vi "OAT Order Cross Spectrum (1x1).vi"(0 "even-angle signal X":cluster{"r0":dbl, "dr":dbl, "Y":dbl[]}={"r0"=0.0, "dr"=1.0, "Y"=[]} {"r0" format="%.2p"; "dr" format="%.2p"; "Y" format="%.2f"}, 1 "even-angle signal Y":cluster{"r0":dbl, "dr":dbl, "Y":dbl[]}={"r0"=0.0, "dr"=1.0, "Y"=[]} {"r0" format="%.2p"; "dr" format="%.2p"; "Y" format="%.2f"}, 2 "window":u32(ring)=1 items=["None"=0, "Hanning"=1, "Hamming"=2, "Blackman-Harris"=3, "Exact Blackman"=4, "Blackman"=5, "Flat Top"=6, "4 Term B-Harris"=7, "7 Term B-Harris"=8, "Low Sidelobe"=9, "Gaussian"=62], 3 "block size":i32=1024 min=2, 4 "view":T6={"dB On (T)"=TRUE, "unwrap phase (F)"=FALSE, "convert to degree (T)"=TRUE}, 5 "error in (no error)":errorcluster, 6 "even-angle channel info X":T1={"channel name"="", "description"="", " channel info"={"sensor sensitivity"=1000.0, "engineering units"=1, "dB reference"=1.0, "custom label"="EU", "weighting filter"=0, "pregain"=0.0}} {"channel info"."pregain" format="%.2f"; "channel info"."weighting filter" items=["Linear", "A-weighting", "B-weighting", "C-weighting", "ITU-R 468-4", "Dolby", "CCITT", "C-message", "Wb", "Wc", "Wd", "We", "Wf", "Wh", "Wj", "Wk", "Wm", "AES17 20 kHz lowpass", "AES17 40 kHz lowpass", "AES17 20 kHz highpass", "AES17 40 kHz highpass"]; "channel info"."dB reference" format="%^.1e"; "channel info"."engineering units" items=["custom..."=0, "V"=1, "A"=21, "C"=30, "pC"=31, "s"=32, "-"=29, "Pa"=2, "N"=20, "g"=3, "m/s^2"=4, "m/s"=5, "m"=6, "mm/s"=12, "mm"=13, "micron/s"=14, "micron"=15, "in/s^2"=7, "in/s"=8, "in"=9, "mil/s"=10, "mil"=11, "rad/s^2"=16, "rad/s"=17, "rad"=18, "deg/s^2"=26, "deg/s"=27, "deg"=28, "RPM"=22, "cycle/s^2"=23, "Hz"=24, "cycle"=25, "strain"=19]; "channel info"."sensor sensitivity" format="%#_5f"}, 7 "averaging parameters":T11={"averaging mode"=enum."No averaging", "weighting mode"=enum."Exponential", "number of averages"=10, "linear mode"=enum."One shot"} {"number of averages" min=1 step=1}, 8 "even-angle channel info Y":T1={"channel name"="", "description"="", " channel info"={"sensor sensitivity"=1000.0, "engineering units"=1, "dB reference"=1.0, "custom label"="EU", "weighting filter"=0, "pregain"=0.0}} {"channel info"."pregain" format="%.2f"; "channel info"."weighting filter" items=["Linear", "A-weighting", "B-weighting", "C-weighting", "ITU-R 468-4", "Dolby", "CCITT", "C-message", "Wb", "Wc", "Wd", "We", "Wf", "Wh", "Wj", "Wk", "Wm", "AES17 20 kHz lowpass", "AES17 40 kHz lowpass", "AES17 20 kHz highpass", "AES17 40 kHz highpass"]; "channel info"."dB reference" format="%^.1e"; "channel info"."engineering units" items=["custom..."=0, "V"=1, "A"=21, "C"=30, "pC"=31, "s"=32, "-"=29, "Pa"=2, "N"=20, "g"=3, "m/s^2"=4, "m/s"=5, "m"=6, "mm/s"=12, "mm"=13, "micron/s"=14, "micron"=15, "in/s^2"=7, "in/s"=8, "in"=9, "mil/s"=10, "mil"=11, "rad/s^2"=16, "rad/s"=17, "rad"=18, "deg/s^2"=26, "deg/s"=27, "deg"=28, "RPM"=22, "cycle/s^2"=23, "Hz"=24, "cycle"=25, "strain"=19]; "channel info"."sensor sensitivity" format="%#_5f"}, 9 "restart averaging? (F)":bool) -> (11 "averaging done?":bool, 12 "new spectrum available?":bool, 13 "averages completed":dbl, 14 "cross spectrum magnitude":T5={"order 0"=0.0, "delta order"=1.0, "magnitude"=[]} {"order 0" format="%.2p"; "delta order" format="%.2p"; "magnitude" format="%.2f"}, 15 "magnitude unit label":string, 16 "cross spectrum phase":T5={"order 0"=0.0, "delta order"=1.0, "magnitude"=[]} {"order 0" format="%.2p"; "delta order" format="%.2p"; "magnitude" format="%.2f"}, 17 "phase unit label":string, 18 "spectrum info":T7={"channel name"="", "description"="", "x-axis units"=0, "spectral info"={"spectrum type"=enum."Power [Magnitude^2]", "linear/dB"=enum."linear", "window"=0, "window size"=0, "FFT size"=0}, "engineering units"=1, "custom label"="", "dB reference [EU]"=0.0, "peak units"=enum."rms", "weighting filter"=0, "spectral density?"=FALSE, "unit label"="", "spectrum skewed?"=FALSE, "complimentary spectrum units"=enum."none"} {"x-axis units" items=["Time (s)"=0, "Frequency-CB (Hz)"=1, "Frequency-CPB (Hz)"=1248, "Frequency-Arbitrary (Hz)"=2357, "Quefrency (s)"=2, "Revolutions (rev)"=3, "Order"=4, "Speed (RPM)"=11, "Speed (rad/s)"=21, "Index"=65535]; "weighting filter" items=["Linear", "A-weighting", "B-weighting", "C-weighting", "ITU-R 468-4", "Dolby", "CCITT", "C-message", "Wb", "Wc", "Wd", "We", "Wf", "Wh", "Wj", "Wk", "Wm", "AES17 20 kHz lowpass", "AES17 40 kHz lowpass", "AES17 20 kHz highpass", "AES17 40 kHz highpass"]; "dB reference [EU]" format="%.2f"; "engineering units" items=["custom..."=0, "V"=1, "A"=21, "C"=30, "pC"=31, "s"=32, "-"=29, "Pa"=2, "N"=20, "g"=3, "m/s^2"=4, "m/s"=5, "m"=6, "mm/s"=12, "mm"=13, "micron/s"=14, "micron"=15, "in/s^2"=7, "in/s"=8, "in"=9, "mil/s"=10, "mil"=11, "rad/s^2"=16, "rad/s"=17, "rad"=18, "deg/s^2"=26, "deg/s"=27, "deg"=28, "RPM"=22, "cycle/s^2"=23, "Hz"=24, "cycle"=25, "strain"=19]; "spectral info"."window" items=["None "=0, "Hanning"=1, "Hamming"=2, "Blackman-Harris"=3, "Exact Blackman"=4, "Blackman"=5, "Flat Top"=6, "4 Term B-Harris "=7, "7 Term B-Harris"=8, "Low Sidelobe"=9, "Force - Exponential"=10, "Gaussian"=62]}, 19 "error out":errorcluster)   [LabVIEW 2017, in "SoundVib_OrderTracking.lvlib"]
doc: "Computes the order power spectrum of an even-angle signal. Wire data to the <B>even-angle signal</B> input to determine the polymorphic instance to use or manually select the instance."
uses:
  <vilib>/addons/Sound and Vibration/Order Analysis/Resample Order Tracking/SoundVib_OrderTracking.lvlib
  <vilib>/addons/_NISVFA/_Shared subVIs/Controls/svc_Spectrum Info.ctl
  <vilib>/addons/_NISVFA/_Shared subVIs/Controls/svc_X-Axis Units.ctl
  <vilib>/addons/_NISVFA/_Shared subVIs/Controls/svc_Spectrum Type.ctl
  <vilib>/addons/_NISVFA/_Shared subVIs/Controls/svc_Engineering Units Text Ring.ctl
  <vilib>/addons/_NISVFA/_Shared subVIs/Controls/svc_Weighting Filter Text Ring.ctl
  <vilib>/addons/_NISVFA/_Shared subVIs/Controls/svc_Complimentary Spectrum Units.ctl
  <vilib>/addons/_NISVFA/_Shared subVIs/Controls/svc_Resampled Channel Info.ctl
  <vilib>/addons/_NISVFA/_Shared subVIs/Controls/svc_Channel Info.ctl
  <vilib>/addons/Sound and Vibration/Order Analysis/Resample Order Tracking/SoundVib_Resampling.lvlib
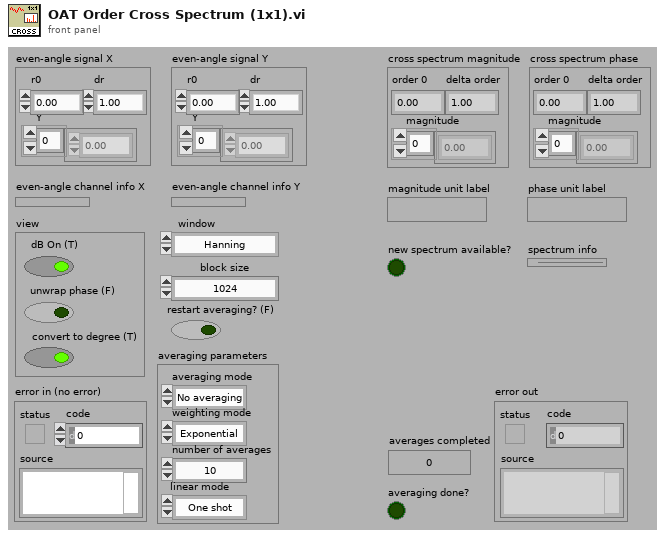
[diagram p1: front panel]
types:
  T1 = typedef "svc_Resampled Channel Info.ctl" = cluster{"channel name":string, "description":string, " channel info":T2}
  T2 = typedef "svc_Channel Info.ctl" = cluster{"sensor sensitivity":dbl, "engineering units":T3, "dB reference":dbl, "custom label":string, "weighting filter":T4, "pregain":dbl}
  T3 = typedef "svc_Engineering Units Text Ring.ctl" = u16
  T4 = typedef "svc_Weighting Filter Text Ring.ctl" = u16
  T5 = cluster{"order 0":dbl, "delta order":dbl, "magnitude":dbl[]}
  T6 = cluster{"dB On (T)":bool, "unwrap phase (F)":bool, "convert to degree (T)":bool}
  T7 = typedef "svc_Spectrum Info.ctl" = cluster{"channel name":string, "description":string, "x-axis units":T8, "spectral info":cluster{"spectrum type":T9, "linear/dB":enum16{"linear", "dB"}, "window":u16, "window size":i32, "FFT size":i32}, "engineering units":T3, "custom label":string, "dB reference [EU]":dbl, "peak units":enum16{"rms", "peak", "peak-peak"}, "weighting filter":T4, "spectral density?":bool, "unit label":string, "spectrum skewed?":bool, "complimentary spectrum units":T10}
  T8 = typedef "svc_X-Axis Units.ctl" = u16
  T9 = typedef "svc_Spectrum Type.ctl" = enum16{"FFT Spectrum [complex]", "Amplitude [Magnitude]", "Power [Magnitude^2]", "Cross Spectrum [complex]", "Frequency Response [Complex]"}
  T10 = typedef "svc_Complimentary Spectrum Units.ctl" = enum16{"none", "radians", "degrees", "cycles", "imaginary"}
  T11 = cluster{"averaging mode":enum16{"No averaging", "Vector averaging", "RMS averaging", "Peak hold"}, "weighting mode":enum16{"Linear", "Exponential"}, "number of averages":u32, "linear mode":enum16{"One shot", "Auto restart"}}
  T12 = cluster{"ignore dt":bool, "ignore t0 continuity":bool, "ignore array length":bool, "ignore channel info":bool, "ignore channel name":bool}
  T13 = enum16{"Cross spectrum", "Frequency response", "Coherent output power"}
  T14 = cluster{"r0":dbl, "dr":dbl, "even angle signal":dbl[]}
  T15 = enum16{"Restart processing", "Continue processing", "Skip processing"}
  T16 = cluster{"complex FFT":cdb[], "power spectrum":dbl[], "averages completed":dbl}
  T17 = enum16{"No averaging", "Vector averaging", "RMS averaging", "Peak hold"}
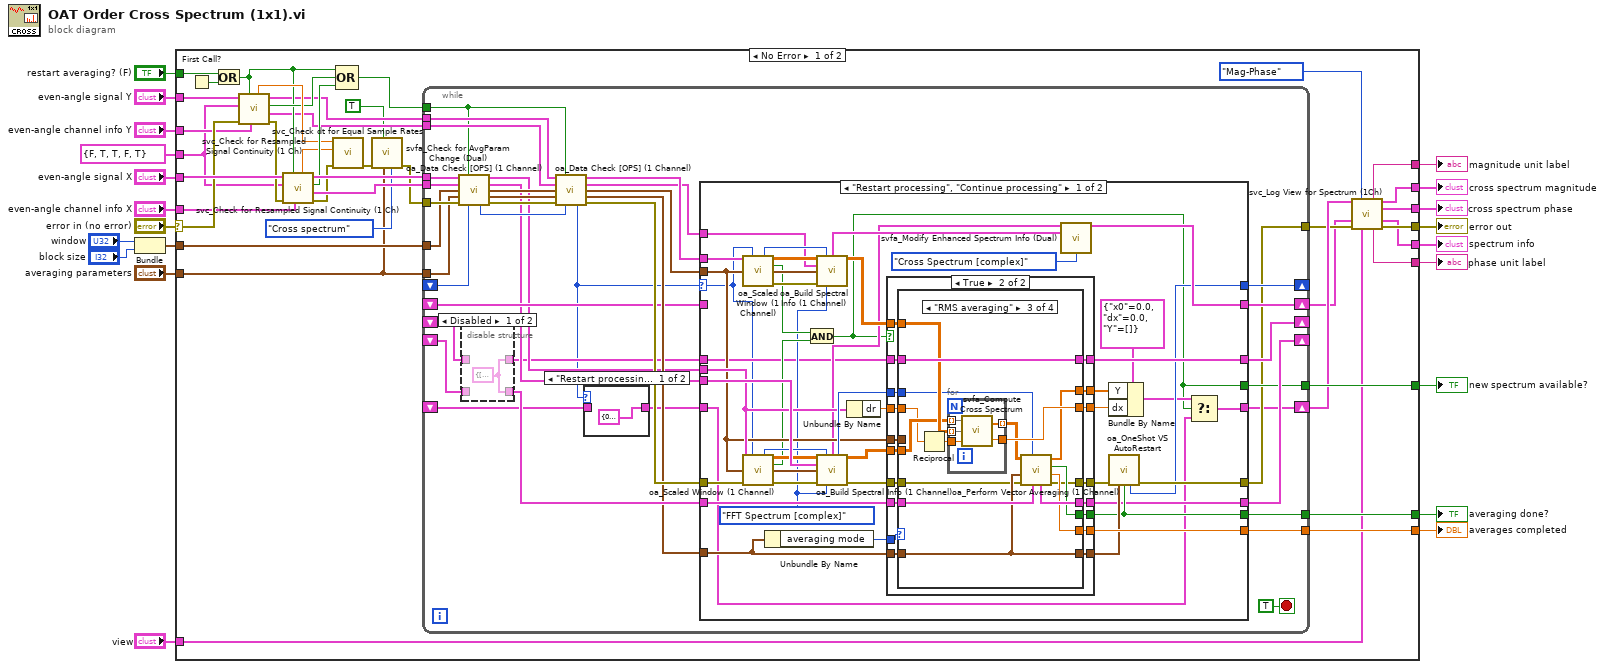
[diagram p0: block diagram]
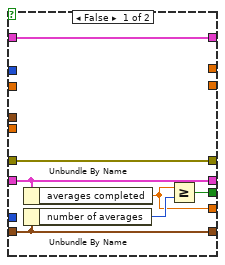
[diagram p4: hidden frame]
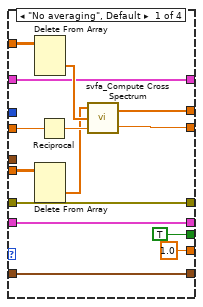
[diagram p5: hidden frame]
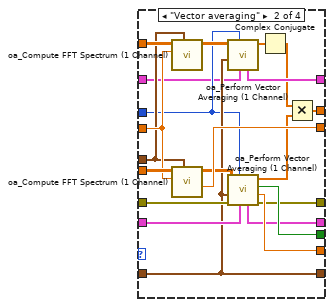
[diagram p6: hidden frame]
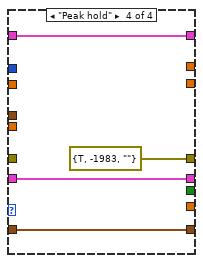
[diagram p7: hidden frame]
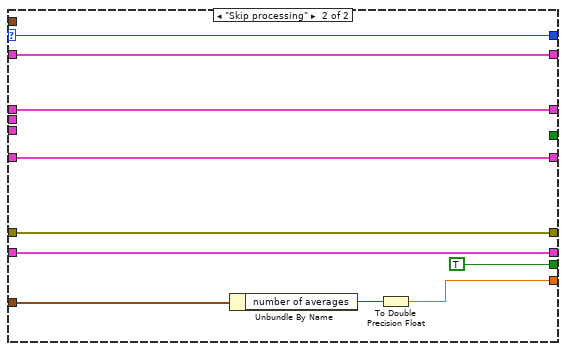
[diagram p8: hidden frame]
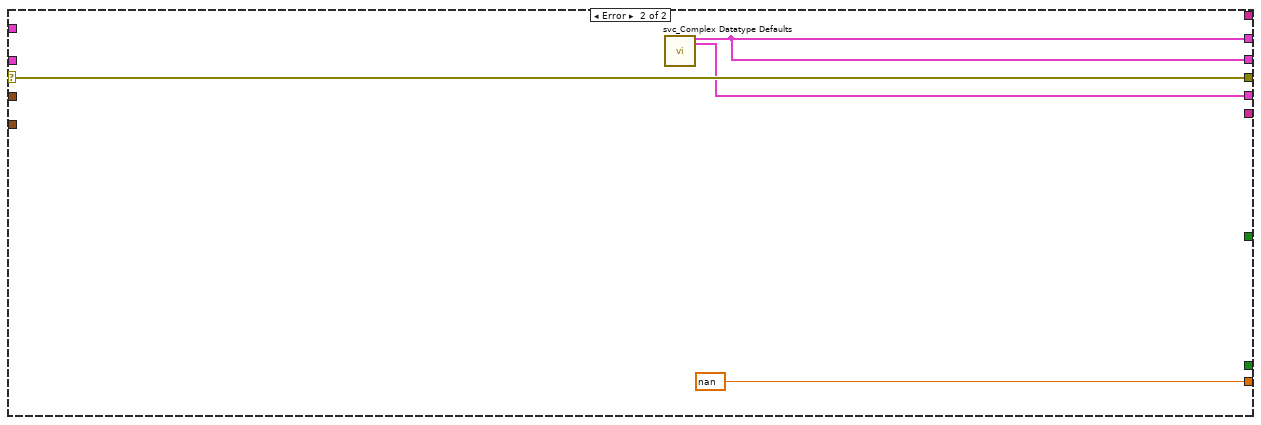
[diagram p9: hidden frame]
diagram:
  n1 = Bundle("window"="window", "block size"="block size") -> (w10:cluster{"window":u32, "block size":i32})  [unwired: 1 in]
  n2 = case shown="No Error" "error in (no error)" {
    selector: "error in (no error)" -> [w50 w249]
    tunnel: "even-angle signal X" -> [w55 _]
    tunnel: "averaging parameters" -> [w37 _]
    tunnel: "restart averaging? (F)" -> [w58 _]
    tunnel: "even-angle channel info X" -> [w38 _]
    tunnel: [w31 w249] -> w18
    tunnel: [w27 w247] -> w17
    tunnel: [w29 w246] -> w16
    tunnel: [w25 _] -> w15
    tunnel: [w61 nan ("averages completed")] -> w14
    tunnel: [w60 _] -> w13
    tunnel: w10 -> [w59 _]
    tunnel: [w56 _] -> w7
    tunnel: "even-angle channel info Y" -> [w39 _]
    tunnel: "even-angle signal Y" -> [w51 _]
    tunnel: T12 {"ignore dt"=FALSE, "ignore t0 continuity"=TRUE, "ignore array length"=TRUE, "ignore channel info"=FALSE, "ignore channel name"=TRUE} ("parameter controls") -> [w35 _]
    tunnel: "view" -> [w30 _]
    tunnel: [w28 w246] -> w2
    tunnel: [w24 _] -> w1
    frame No Error {
      n3 = First Call?() -> (First Call?: T/F=w57:bool)
      n4 = Or(x=w58, y=w57) -> (x .or. y?=w44:bool)
      n5 = call <vilib>:"svc_Check for Resampled Signal Continuity (1 Ch).vi"("even angle channel info"=w39, "restart averaging (F)"=w44, "error in (no error)"=w50, "parameter controls"=w35, "even angle signal"=w51) -> ("error out"=w49:errorcluster, "dup even angle channel info"=w40:T1, "waveform parameter changed"=w45:bool, "dup even angle signal"=w41:T14, "dt"=w47:dbl)  [unwired: 1 in, 1 out]
      n6 = call <vilib>:"svc_Check for Resampled Signal Continuity (1 Ch).vi"("even angle channel info"=w38, "restart averaging (F)"=w44, "error in (no error)"=w49, "parameter controls"=w35, "even angle signal"=w55) -> ("error out"=w46:errorcluster, "dup even angle channel info"=w53:T1, "waveform parameter changed"=w52:bool, "dup even angle signal"=w54:T14, "dt"=w48:dbl)  [unwired: 1 in, 1 out]
      n7 = call <vilib>:"svc_Check dt for Equal Sample Rates.vi"("error in (no error)"=w46, "dt Y"=w48, "dt X"=w47) -> ("error out"=w42:errorcluster)  [unwired: 7 in, 1 out]
      n8 = Compound Arithmetic op=OR(w44, w45, w52) -> (w23:bool)
      n9 = call <vilib>:"svfa_Check for AvgParam Change (Dual).vi"("measurement"=T13."Cross spectrum", "averaging parameters"=w37, "restart averaging (F)"=TRUE, "error in (no error)"=w42) -> ("error out"=w36:errorcluster)  [unwired: 6 in, 1 out]
      n10 = while {
        tunnel: w54 -> [w99]
        tunnel: w37 -> [w78]
        tunnel: w23 -> [w66]
        tunnel: w53 -> [w96]
        tunnel: [w67] -> w32
        tunnel: [w87] -> w61
        tunnel: [w86] -> w60
        shift-right: [w88] -> _
        shift-left: _ -> [w97]
        tunnel: w59 -> [w80]
        tunnel: [w81] -> w56
        tunnel: w36 -> [w95]
        tunnel: w41 -> [w94]
        tunnel: w40 -> [w93]
        shift-right: [w85] -> _
        shift-left: _ -> [w84]
        shift-right: [w76] -> w26
        shift-left: _ -> [w75]
        shift-right: [w68] -> _
        shift-left: _ -> [w70]
        shift-right: [w62] -> w33
        shift-left: _ -> [w64]
        stop <- TRUE stop-if-true
        n11 = call <vilib>:"oa_Data Check [OPS] (1 Channel).vi"("resampled signal"=w99, "restart averaging (F)"=w66, "resampled channel info"=w96, "spectrum settings"=w80, "averaging parameters"=w78, "error in (no error)"=w95, "processing control in"=w97) -> ("dup resampled signal"=w71:cluster{"r0":dbl, "dr":dbl, "Y":dbl[]}, "dup resampled channel info"=w72:T1, "dup spectrum settings"=w90:cluster{"window type":u32, "block size":i32}, "dup averaging parameters"=w91:T11, "processing control out"=w89:T15, "error out"=w92:errorcluster)  [unwired: 3 in]
        n12 = disable-structure shown="Disabled" {
          disable-tunnel: [w102 w104] -> w83
          disable-tunnel: w84 -> [_ w104]
          disable-tunnel: w70 -> [_ w103]
          disable-tunnel: [w102 w103] -> w69
          frame Disabled {
            w102 = T16 {"complex FFT"=[], "power spectrum"=[], "averages completed"=0.0} ("averaging state info out")
          }
          frame Enabled {
          }
        }
        n13 = call <vilib>:"oa_Data Check [OPS] (1 Channel).vi"("resampled signal"=w94, "restart averaging (F)"=w66, "resampled channel info"=w93, "spectrum settings"=w90, "averaging parameters"=w91, "error in (no error)"=w92, "processing control in"=w89) -> ("dup resampled signal"=w74:cluster{"r0":dbl, "dr":dbl, "Y":dbl[]}, "dup resampled channel info"=w73:T1, "dup spectrum settings"=w79:cluster{"window type":u32, "block size":i32}, "dup averaging parameters"=w77:T11, "processing control out"=w65:T15, "error out"=w82:errorcluster)  [unwired: 3 in]
        n14 = case shown="\"Restart processing\"" w65 {
          tunnel: w64 -> [_ w101]
          tunnel: [cluster{dbl, "df [Hz]":dbl, "Y out":cdb[]} {0.0, "df [Hz]"=0.0, "Y out"=[]} w101] -> w63
          frame "Restart processing" {
          }
          frame Default {
          }
        }
        n15 = case shown="\"Restart processing\", \"Continue processing\"" w65 {
          selector: w65 -> [w106 w239]
          tunnel: w71 -> [w141 _]
          tunnel: w82 -> [w150 w244]
          tunnel: w79 -> [w126 _]
          tunnel: w72 -> [w147 _]
          tunnel: w77 -> [w131 w242]
          tunnel: [w119 w245] -> w76
          tunnel: w75 -> [_ w245]
          tunnel: [w136 w244] -> w67
          tunnel: [w139 w240] -> w87
          tunnel: [w134 TRUE ("averaging done")] -> w86
          tunnel: w63 -> [w107 w236]
          tunnel: [w111 w239] -> w88
          tunnel: [w133 w238] -> w85
          tunnel: w83 -> [w132 w238]
          tunnel: [w108 _] -> w81
          tunnel: w74 -> [w125 _]
          tunnel: w73 -> [w124 _]
          tunnel: w69 -> [w115 w237]
          tunnel: [w114 w237] -> w68
          tunnel: [w109 w236] -> w62
          frame "Restart processing", "Continue processing" {
            w121 = svc_Spectrum_Type."FFT Spectrum [complex]" ("spectrum type")
            n16 = call <vilib>:"oa_Scaled Window (1 Channel).vi"("resampled signal"=w125, "processing control in"=w106, "spectrum settings"=w126) -> ("dup processing control"=w127:T15, "Y"=w130:dbl[][], "new spectrum available?"=w123:bool, "spectrum settings"=w129:cluster{"window type":u32, "block size":i32}, "error out"=w128:errorcluster)  [unwired: 8 in]
            n17 = call <vilib>:"oa_Scaled Window (1 Channel).vi"("resampled signal"=w141, "processing control in"=w106, "spectrum settings"=w126, "error in"=w150) -> ("dup processing control"=w146:T15, "Y"=w144:dbl[][], "new spectrum available?"=w122:bool, "spectrum settings"=w148:cluster{"window type":u32, "block size":i32}, "error out"=w149:errorcluster)  [unwired: 7 in]
            n18 = Unbundle By Name(w131) -> ("averaging mode"=w145:T17)
            n19 = And(x=w123, y=w122) -> (x .and. y?=w108:bool)
            n20 = call <vilib>:"oa_Build Spectral Info (1 Channel).vi"("spectra in"=w130, "processing control in"=w127, "resampled channel info"=w124, "spectrum settings"=w129, "error in"=w128, "spectrum type"=w121) -> ("spectrum info"=w120:T7, "spectra out"=w117:dbl[][])  [unwired: 6 in, 2 out]
            n21 = call <vilib>:"oa_Build Spectral Info (1 Channel).vi"("spectra in"=w144, "processing control in"=w146, "resampled channel info"=w147, "spectrum settings"=w148, "error in"=w149, "spectrum type"=w121) -> ("spectrum info"=w116:T7, "dup processing control"=w142:T15, "spectra out"=w105:dbl[][], "error out"=w143:errorcluster)  [unwired: 6 in]
            n22 = Unbundle By Name(w141) -> ("dr"=w140:dbl)
            n23 = case shown="True" w108 {
              tunnel: w145 -> [_ w175]
              tunnel: w105 -> [_ w174]
              tunnel: w143 -> [w156 w173]
              tunnel: w142 -> [_ w172]
              tunnel: w140 -> [_ w171]
              tunnel: [w151 w170] -> w139
              tunnel: [_ w169] -> w138
              tunnel: [_ w168] -> w112
              tunnel: [w156 w167] -> w137
              tunnel: [w154 w166] -> w135
              tunnel: [w152 w165] -> w134
              tunnel: [w155 w164] -> w133
              tunnel: w132 -> [w155 w163]
              tunnel: w131 -> [w154 w162]
              tunnel: w126 -> [_ w161]
              tunnel: w117 -> [_ w160]
              tunnel: w115 -> [w157 w159]
              tunnel: [w157 w158] -> w114
              frame False {
                n24 = Unbundle By Name(w155) -> ("averages completed"=w151:dbl)
                n25 = Unbundle By Name(w154) -> ("number of averages"=w153:u32)
                n26 = Greater Or Equal?(x=w151, y=w153) -> (x >= y?=w152:bool)
              }
              frame True {
                n27 = case shown="\"RMS averaging\"" w175 {
                  tunnel: w174 -> [w182 w210 w224 _]
                  tunnel: w173 -> [w189 w208 w214 _]
                  tunnel: w172 -> [_ w196 w212 _]
                  tunnel: w171 -> [w184 w199 w223 _]
                  tunnel: [w180 w192 w217 _] -> w169
                  tunnel: [w189 w204 w213 errorcluster {"status"=TRUE, "code"=-1983, "source"=""} ("error out")] -> w167
                  tunnel: w162 -> [w186 w200 w218 w233]
                  tunnel: [1.0 ("averages completed") w205 w215 _] -> w170
                  tunnel: [TRUE ("averaging done") w206 w216 _] -> w165
                  tunnel: [w179 w209 w222 _] -> w168
                  tunnel: [w186 w200 w218 w233] -> w166
                  tunnel: [w185 w202 w220 w234] -> w164
                  tunnel: w163 -> [w185 w203 w221 w234]
                  tunnel: w161 -> [_ w198 _ _]
                  tunnel: w160 -> [w183 w201 w225 _]
                  tunnel: w159 -> [w176 w195 w226 w235]
                  tunnel: [w176 w194 w226 w235] -> w158
                  frame "No averaging", Default {
                    n28 = Delete From Array(array=w183) -> (deleted portion=w178:dbl[])  [unwired: 3 in, 1 out]
                    n29 = Delete From Array(array=w182) -> (deleted portion=w177:dbl[])  [unwired: 3 in, 1 out]
                    n30 = Reciprocal(x=w184) -> (1/x=w181:dbl)
                    n31 = call <vilib>:"svfa_Compute Cross Spectrum.vi"("sampling frequency [Hz]"=w181, "signal Y [EUy]"=w178, "signal X [EUx]"=w177) -> ("df [Hz]"=w179:dbl, "cross spectrum [EUx EUy rms]"=w180:cdb[])
                  }
                  frame "Vector averaging" {
                    n32 = call <vilib>:"oa_Compute FFT Spectrum (1 Channel).vi"("spectrum settings"=w198, "dr"=w199, "Y"=w201) -> ("one-sided FFT spectrum"=w197:cdb[][])  [unwired: 7 in, 1 out]
                    n33 = call <vilib>:"oa_Compute FFT Spectrum (1 Channel).vi"("spectrum settings"=w198, "dr"=w199, "Y"=w210) -> ("df"=w209:dbl, "one-sided FFT spectrum"=w207:cdb[][])  [unwired: 7 in]
                    n34 = call <vilib>:"oa_Perform Vector Averaging (1 Channel).vi"("averaging state info in"=w195, "processing control in"=w196, "averaging parameters"=w200, "Y"=w197) -> ("Y out"=w191:cdb[], "averaging state info out"=w194:T16)  [unwired: 3 in, 3 out]
                    n35 = call <vilib>:"oa_Perform Vector Averaging (1 Channel).vi"("averaging state info in"=w203, "processing control in"=w196, "error in (no error)"=w208, "averaging parameters"=w200, "Y"=w207) -> ("error out"=w204:errorcluster, "averages completed"=w205:dbl, "averaging done"=w206:bool, "Y out"=w193:cdb[], "averaging state info out"=w202:T16)  [unwired: 2 in]
                    n36 = Complex Conjugate(1:w191) -> (0:w190:cdb[])
                    n37 = Multiply(x=w190, y=w193) -> (x*y=w192:cdb[])
                  }
                  frame "RMS averaging" {
                    n38 = Reciprocal(x=w223) -> (1/x=w211:dbl)
                    n39 = for {
                      tunnel: w225 -> [w231] mode=indexing
                      tunnel: w224 -> [w230] mode=indexing
                      tunnel: w211 -> [w229]
                      tunnel: [w228] -> w219 mode=indexing
                      tunnel: [w227] -> w222
                      n40 = call <vilib>:"svfa_Compute Cross Spectrum.vi"("sampling frequency [Hz]"=w229, "signal Y [EUy]"=w231, "signal X [EUx]"=w230) -> ("df [Hz]"=w227:dbl, "cross spectrum [EUx EUy rms]"=w228:cdb[])
                    }
                    n41 = call <vilib>:"oa_Perform Vector Averaging (1 Channel).vi"("averaging state info in"=w221, "processing control in"=w212, "error in (no error)"=w214, "averaging parameters"=w218, "Y"=w219) -> ("error out"=w213:errorcluster, "averages completed"=w215:dbl, "averaging done"=w216:bool, "Y out"=w217:cdb[], "averaging state info out"=w220:T16)  [unwired: 2 in]
                  }
                  frame "Peak hold" {
                  }
                }
              }
            }
            n42 = call <vilib>:"svfa_Modify Enhanced Spectrum Info (Dual).vi"("spectrum info X"=w116, "spectrum info Y"=w120, "spectrum type"=svc_Spectrum_Type."Cross Spectrum [complex]") -> ("spectrum info"=w119:T7)  [unwired: 10 in, 2 out]
            n43 = Bundle By Name(cluster=cluster{"x0":dbl, "dx":dbl, "Y":cdb[]} {"x0"=0.0, "dx"=0.0, "Y"=[]}, "Y"=w138, "dx"=w112) -> (w110:cluster{"x0":dbl, "dx":dbl, "Y":cdb[]})
            n44 = call <vilib>:"oa_OneShot VS AutoRestart.vi"("error in (no error)"=w137, "averaging parameters"=w135, "averaging done"=w134) -> ("processing control out"=w111:T15, "error out"=w136:errorcluster)  [unwired: 11 in]
            n45 = Select(t=w110, s=w108, f=w107) -> (s? t:f=w109:cluster{"x0":dbl, "df [Hz]":dbl, "Y out":cdb[]})
          }
          frame "Skip processing" {
            n46 = Unbundle By Name(w242) -> ("number of averages"=w241:u32)
            n47 = To Double Precision Float(number=w241) -> (double precision float=w240:dbl)
          }
        }
      }
      n48 = call <vilib>:"svc_Log View for Spectrum (1Ch).vi"("complex spectrum"=w33, "View"=enum16{"Mag-Phase", "Real-Imaginary"}."Mag-Phase", "spectrum info in"=w26, "error in (no error)"=w32, "view"=w30) -> ("unit label [mag or real]"=w25:string, "magnitude or real"=w29:cluster{"f0":dbl, "df":dbl, dbl[]}, "phase or imag"=w28:cluster{"f0":dbl, "df":dbl, dbl[]}, "spectrum info out"=w27:T7, "unit label [phase or imag]"=w24:string, "error out"=w31:errorcluster)  [unwired: 5 in]
    }
    frame Error {
      n49 = call <vilib>:"svc_Complex Datatype Defaults.vi"() -> ("empty spectrum"=w246:cluster{"f0":dbl, "df":dbl, "magnitude":dbl[]}, "dead spectrum info"=w247:T7)  [unwired: 11 in, 7 out]
    }
  }
  "cross spectrum magnitude" <- w16
  "magnitude unit label" <- w15
  "error out" <- w18
  "averaging done?" <- w13
  "averages completed" <- w14
  "spectrum info" <- w17
  "new spectrum available?" <- w7
  "cross spectrum phase" <- w2
  "phase unit label" <- w1
